vi "speedline graph format.vi"(11 "Cluster in":T1={"rigChannels"=[], "rigUnits"=[], "logging"=FALSE, "chartRef"=refnum, "dataTableRef"=refnum, "channelCount"=0, "trendIndex"=0, "channels"={"massflow"=0, "PR"=0, "recircTemp"=0}, "History"={"speedlines"=[], "liveTail"={"mDot"=[], "pRatio"=[]}, "current"={"mDot"=0.0, "pRatio"=0.0}, "insertPoint"=0, "tempHistory"=[]}, "filter"=FALSE, "filterLength"=0, "tableUpdate"=0, "limitValues"=[[0.0, 45000.0], [0.0, 100.0], [0.0, 100.0], [10.0, 100.0], [0.0, 100.0], [10.0, 35.0], [0.0, 100.0], [0.0, 100.0], [99000.0, 300000.0], [-5000.0, 5000.0], [99000.0, 300000.0], [-0.01, 0.3], [-0.01, 4.5], [-0.1, 100.0], [1.0, 8.0], [1.0, 5.0], [0.0, 100.0], [0.0, 100.0], [0.0, 100.0], [-100.0, 45000.0], [-0.1, 1.0], [0.8, 2.0], [90000.0, 110000.0], [15.0, 35.0], [0.0, 0.0], [0.0, 0.0], [0.0, 0.0], [0.0, 0.0]]}) -> ()   [LabVIEW 2018]
uses:
  custom sub vis/speedlineData.ctl
types:
  T1 = typedef "speedlineData.ctl" = cluster{"rigChannels":string[], "rigUnits":string[], "logging":bool, "chartRef":refnum<vi>, "dataTableRef":refnum<vi>, "channelCount":i32, "trendIndex":i32, "channels":cluster{"massflow":i32, "PR":i32, "recircTemp":i32}, "History":cluster{"speedlines":cluster{"mDot":dbl[], "pRatio":dbl[]}[], "liveTail":cluster{"mDot":dbl[], "pRatio":dbl[]}, "current":cluster{"mDot":dbl, "pRatio":dbl}, "insertPoint":i32, "tempHistory":dbl[][]}, "filter":bool, "filterLength":i32, "tableUpdate":i16, "limitValues":dbl[][]}
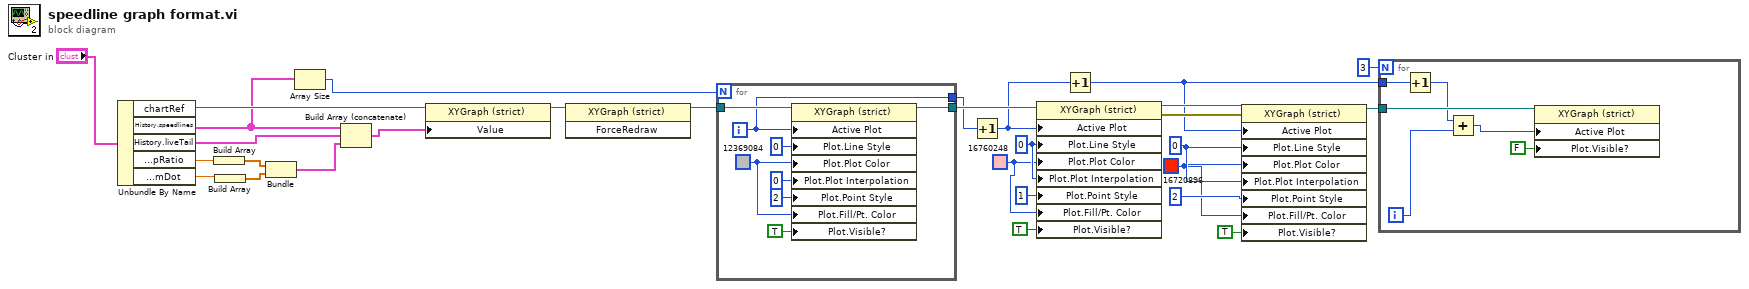
[diagram p0: block diagram]
diagram:
  w6 = u32 16720896 ("Plot.Plot Color")
  w9 = u8 0 ("Plot.Line Style")
  w7 = u32 16760248 ("Plot.Plot Color")
  w14 = u8 0 ("Plot.Line Style")
  n1 = Unbundle By Name("Cluster in") -> ("chartRef"=w28:refnum<vi>, "History.speedlines"=w20:cluster{"mDot":dbl[], "pRatio":dbl[]}[], "History.liveTail"=w21:cluster{"mDot":dbl[], "pRatio":dbl[]}, "History.current.pRatio"=w27:dbl, "History.current.mDot"=w26:dbl)
  n2 = Build Array(w27) -> (w25:dbl[])
  n3 = Build Array(w26) -> (w24:dbl[])
  n4 = Bundle(w25, w24) -> (w23:cluster{dbl[], dbl[]})  [unwired: 1 in]
  n5 = Array Size(array=w20) -> (size(s)=w17:i32)
  n6 = Build Array (concatenate)(w20, w21, w23) -> (w22:cluster{"mDot":dbl[], "pRatio":dbl[]}[])
  n7 = property class="XYGraph (strict)"(reference=w28, "Value"=w22) -> (reference out=w19:refnum<vi>)  [unwired: 1 in, 1 out]
  n8 = invoke class="XYGraph (strict)" method="ForceRedraw"(reference=w19) -> (reference out=w18:refnum<vi>)  [unwired: 2 in, 2 out]
  n9 = for {
    N: w17 -> [_]
    tunnel: w18 -> [w37]
    tunnel: [w35] -> w15
    tunnel: [w32] -> w16
    i -> [w35]
    w31 = u32 12369084 ("Plot.Plot Color")
    n10 = property class="XYGraph (strict)"(reference=w37, "Active Plot"=w35, "Plot.Line Style"=u8 0, "Plot.Plot Color"=w31, "Plot.Plot Interpolation"=u8 0, "Plot.Point Style"=u8 2, "Plot.Fill/Pt. Color"=w31, "Plot.Visible?"=TRUE ("Plot.Visible")) -> (reference out=w32:refnum<vi>)  [unwired: 1 in, 1 out]
  }
  n11 = Increment(x=w15) -> (x+1=w10:i32)
  n12 = property class="XYGraph (strict)"(reference=w16, "Active Plot"=w10, "Plot.Line Style"=w14, "Plot.Plot Color"=w7, "Plot.Plot Interpolation"=w14, "Plot.Point Style"=u8 1, "Plot.Fill/Pt. Color"=w7, "Plot.Visible?"=TRUE ("Plot.Visible")) -> (reference out=w12:refnum<vi>, error out=w11:errorcluster)  [unwired: 1 in]
  n13 = Increment(x=w10) -> (x+1=w4:i32)
  n14 = property class="XYGraph (strict)"(reference=w12, error in=w11, "Active Plot"=w4, "Plot.Line Style"=w9, "Plot.Plot Color"=w6, "Plot.Plot Interpolation"=w9, "Plot.Point Style"=u8 2, "Plot.Fill/Pt. Color"=w6, "Plot.Visible?"=TRUE ("Plot.Visible")) -> (reference out=w5:refnum<vi>)  [unwired: 1 out]
  n15 = for {
    N: 3 -> [_]
    tunnel: w5 -> [w43]
    tunnel: w4 -> [w41]
    i -> [w39]
    n16 = Increment(x=w41) -> (x+1=w40:i32)
    n17 = Add(x=w40, y=w39) -> (x+y=w38:i32)
    n18 = property class="XYGraph (strict)"(reference=w43, "Active Plot"=w38, "Plot.Visible?"=FALSE ("Plot.Visible")) -> ()  [unwired: 1 in, 2 out]
  }
